vi "OBIS Test Remote Commands.vi"() -> ()   [LabVIEW 8.6]
uses:
  <vilib>/Instr/_visa.llb/VISA Configure Serial Port (Instr).vi
panel:
  in  "Send":bool
  in  "stop":bool
  out "read from laser":string
  in  "write to laser":string
  in  "VISA resource name":refnum<visa-resource-name>
  # "This VI can be used to send and receive any of the ASCII commands that are printed in the OBIS user manual.  The VISA resouce name should be set prior to running this VI.  The VISA resouce should match the COM port number that the laser is associated with.  To check this COM port number, you can look in Device Manager under the Ports category for the laser."
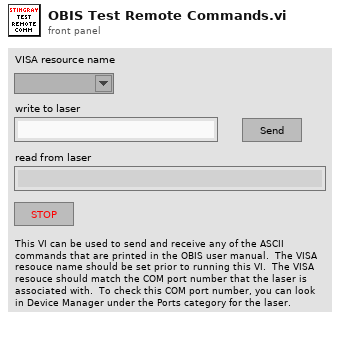
[diagram p1: front panel]
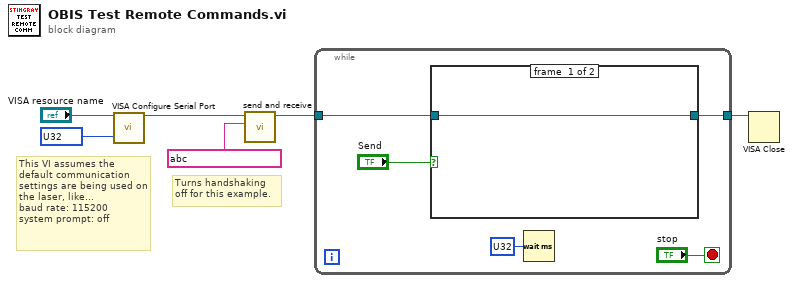
[diagram p0: block diagram]
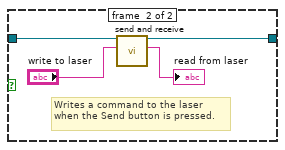
[diagram p2: hidden frame]
diagram:
  # "Turns handshaking\noff for this example."
  # "This VI assumes the default communication settings are being used on the laser, like...\nbaud rate: 115200\nsystem prompt: off"
  n1 = call-poly "VISA Configure Serial Port"("VISA resource name"="VISA resource name", "baud rate (9600)"=u32 ?) -> ("VISA resource name out"=w2:refnum<visa-resource-name>)  [unwired: 12 in, 1 out]
  n2 = call "send and receive.vi"("write to laser"=string ?, "VISA resource name"=w2) -> ("VISA resource name out"=w1:refnum<visa-resource-name>)  [unwired: 8 in, 1 out]
  n3 = while {
    tunnel: w1 -> [w10]
    tunnel: [w8] -> w4
    stop <- "stop" stop-if-true
    n4 = case shown="True" "Send" {
      tunnel: w10 -> [w12 w16]
      tunnel: [w12 w14] -> w8
      frame #0 {
      }
      frame #1 {
        # "Writes a command to the laser when the Send button is pressed."
        n5 = call "send and receive.vi"("write to laser"="write to laser", "VISA resource name"=w16) -> ("read from laser"=→"read from laser":string, "VISA resource name out"=w14:refnum<visa-resource-name>)  [unwired: 8 in]
      }
    }
    n6 = Wait (ms)(milliseconds to wait=u32 ?) -> ()  [unwired: 1 out]
  }
  n7 = VISA Close(VISA resource name=w4) -> ()  [unwired: 1 in, 1 out]
